vi "Switch Disconnect.vi"(8 "error in (no error)":errorcluster, 10 "Channels Connected":string[](array[string]), 11 "Switch Refs":refnum<k15>[](array[refnum])) -> (0 "error out":errorcluster)   [LabVIEW 2019]
uses:
  <instrlib>/niSwitch/niSwitch.llb/niSwitch Disconnect Channels (Multiple).vi
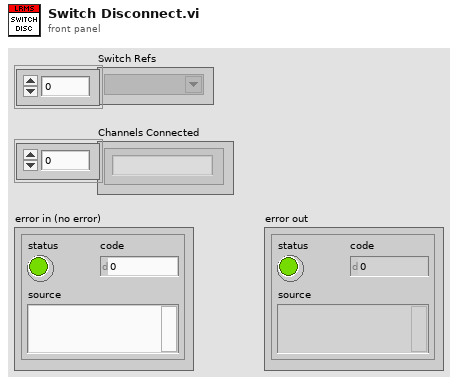
[diagram p1: front panel]
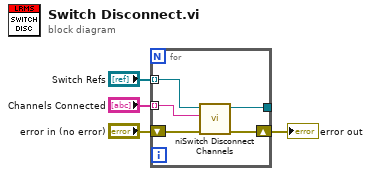
[diagram p0: block diagram]
diagram:
  n1 = for {
    tunnel: "Switch Refs" -> [w9] mode=indexing
    shift-right: [w6] -> w1
    shift-left: "error in (no error)" -> [w8]
    tunnel: [w7] -> _
    tunnel: "Channels Connected" -> [w5] mode=indexing
    n2 = call-poly <instrlib>:"niSwitch Disconnect Channels.vi"("error in (no error)"=w8, "disconnection list"=w5, "instrument handle"=w9) -> ("error out"=w6:errorcluster, "instrument handle out"=w7:refnum<k15>)  [unwired: 7 in]
  }
  "error out" <- w1
